vi "Write RTM Activated Msg.vi"(10 "Interface.lvlib:RTM Activated Msg.lvclass":refnum<class "RTM Activated Msg.lvclass">, 11 "Interface in":refnum<class "Interface.lvclass">) -> (3 "Interface out":refnum<class "Interface.lvclass">)   [LabVIEW 2015, in "Interface.lvlib" / "Interface.lvclass"]
uses:
  Interface.lvclass
  Interface Messages/RTM Activated Msg/RTM Activated Msg.lvclass
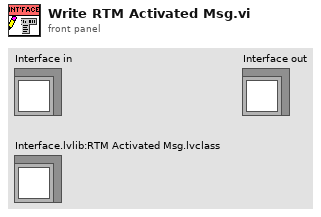
[diagram p1: front panel]
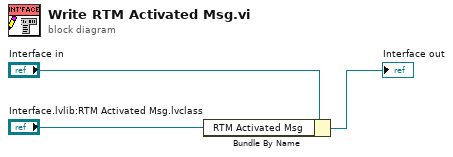
[diagram p0: block diagram]
diagram:
  n1 = Bundle By Name(cluster="Interface in", "RTM Activated Msg"="Interface.lvlib:RTM Activated Msg.lvclass") -> (→"Interface out":refnum<class "Interface.lvclass">)
